vi "StreamTransmitInstrument.vi"() -> ()   [LabVIEW 2018]
panel:
  in  "stop":bool
  out "error out":errorcluster
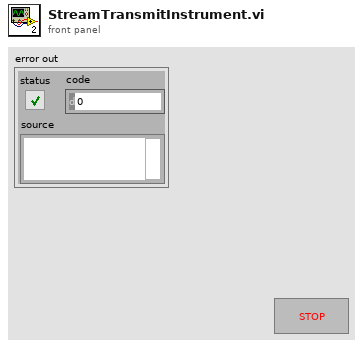
[diagram p1: front panel]
types:
  T1 = cluster{"ID":u32, "Address":string, "Service Name 1":string, "Service Name 2":string, "queue TX":refnum<queue>, "queue RX":refnum<queue>, "Port 1":u32, "Port 2":u32}
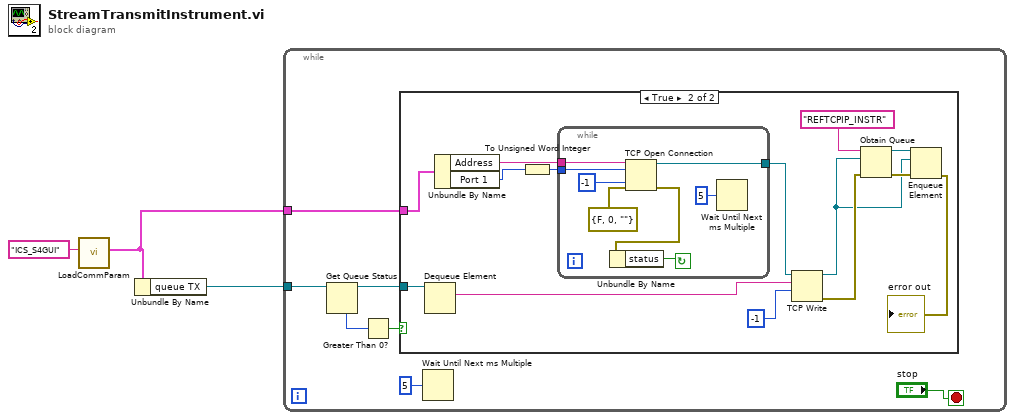
[diagram p0: block diagram]
diagram:
  n1 = call "LoadCommParam.vi"("section name"="ICS_S4GUI") -> ("output cluster"=w1:T1)  [unwired: 10 in]
  n2 = Unbundle By Name(w1) -> ("queue TX"=w2:refnum<queue>)
  n3 = while {
    tunnel: w2 -> [w9]
    tunnel: w1 -> [w4]
    stop <- "stop" stop-if-true
    n4 = Get Queue Status(queue=w9) -> (queue out=w6:refnum<queue>, # elements in queue=w8:i32)  [unwired: 2 in, 6 out]
    n5 = Greater Than 0?(x=w8) -> (x > 0?=w7:bool)
    n6 = case shown="True" w7 {
      tunnel: w6 -> [_ w24]
      tunnel: w4 -> [_ w22]
      frame False {
      }
      frame True {
        n7 = Dequeue Element(queue=w24) -> (element=w23:string)  [unwired: 2 in, 3 out]
        n8 = Unbundle By Name(w22) -> ("Address"=w12:string, "Port 1"=w11:u32)
        n9 = To Unsigned Word Integer(number=w11) -> (unsigned 16bit integer=w13:u16)
        n10 = while {
          tunnel: [w32] -> w21
          tunnel: w13 -> [w31]
          tunnel: w12 -> [w30]
          stop <- w26 continue-if-true
          n11 = TCP Open Connection(address=w30, remote port or service name=w31, timeout ms (60000)=-1, error in (no error)=errorcluster {"status"=FALSE, "code"=0, "source"=""}) -> (connection ID=w32:refnum<k5>, error out=w27:errorcluster)  [unwired: 1 in]
          n12 = Unbundle By Name(w27) -> ("status"=w26:bool)
          n13 = Wait Until Next ms Multiple(millisecond multiple=u32 5) -> ()  [unwired: 1 out]
        }
        n14 = TCP Write(connection ID=w21, data in=w23, 9:-1 ("timeout ms (25000)")) -> (connection ID out=w17:refnum<k5>, error out=w19:errorcluster)  [unwired: 1 in, 1 out]
        n15 = Obtain Queue(name (unnamed)="REFTCPIP_INSTR", element data type=w17, error in (no error)=w19) -> (queue out=w16:refnum<queue>, error out=w18:errorcluster)  [unwired: 2 in, 1 out]
        n16 = Enqueue Element(queue=w16, element=w17, error in (no error)=w18) -> (error out=→"error out":errorcluster)  [unwired: 1 in, 2 out]
      }
    }
    n17 = Wait Until Next ms Multiple(millisecond multiple=u32 5) -> ()  [unwired: 1 out]
  }
